vi "ConfigMeasurement.vi"(8 "error in (no error)":errorcluster, 11 "HP3458aDMM in":refnum<class "HP3458aDMM.lvclass">) -> (0 "error out":errorcluster, 3 "HP3458aDMM out":refnum<class "HP3458aDMM.lvclass">)   [LabVIEW 2014, in "SamplerPlugins.lvlib" / "HP3458aDMM.lvclass"]
uses:
  HP3458aDMM.lvclass
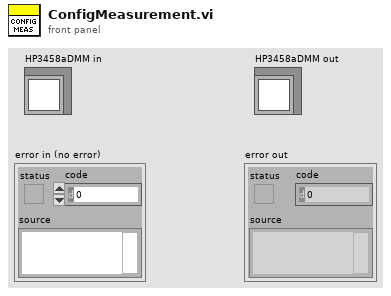
[diagram p1: front panel]
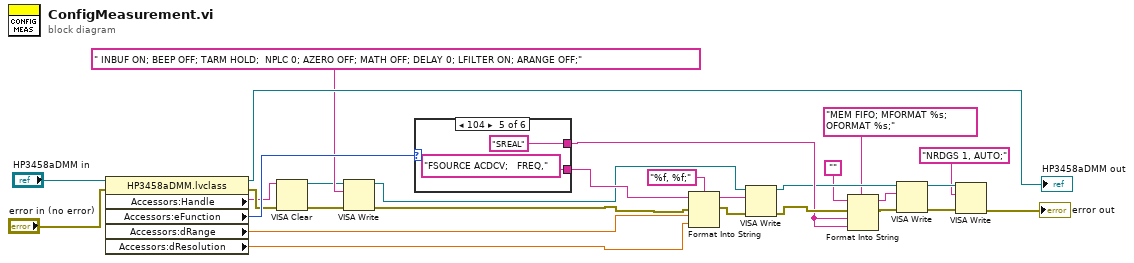
[diagram p0: block diagram]
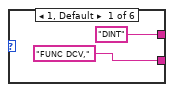
[diagram p2: hidden frame]
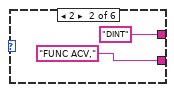
[diagram p3: hidden frame]
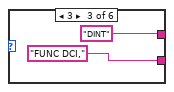
[diagram p4: hidden frame]
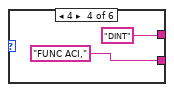
[diagram p5: hidden frame]
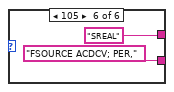
[diagram p6: hidden frame]
diagram:
  n1 = property class="HP3458aDMM.lvclass"(reference="HP3458aDMM in", error in="error in (no error)") -> (reference out=→"HP3458aDMM out":refnum<class "HP3458aDMM.lvclass">, error out=w22:errorcluster, "Accessors:Handle"=w21:string, "Accessors:eFunction"=w23:u16, "Accessors:dRange"=w26:dbl, "Accessors:dResolution"=w25:dbl)
  n2 = VISA Clear(VISA resource name=w21, error in (no error)=w22) -> (VISA resource name out=w12:refnum<visa-resource-name>, error out=w14:errorcluster)
  n3 = VISA Write(VISA resource name=w12, write buffer=" INBUF ON; BEEP OFF; TARM HOLD;  NPLC 0; AZERO OFF; MATH OFF; DELAY 0; LFILTER ON; ARANGE OFF;" ("string"), error in (no error)=w14) -> (VISA resource name out=w11:refnum<visa-resource-name>, error out=w13:errorcluster)  [unwired: 1 out]
  n4 = case shown="104" w23 {
    tunnel: ["FUNC DCV," "FUNC ACV," "FUNC DCI," "FUNC ACI," "FSOURCE ACDCV;   FREQ," "FSOURCE ACDCV; PER,"] -> w16
    tunnel: ["DINT" "DINT" "DINT" "DINT" "SREAL" "SREAL"] -> w8
    frame 1, Default {
    }
    frame 2 {
    }
    frame 3 {
    }
    frame 4 {
    }
    frame 104 {
    }
    frame 105 {
    }
  }
  n5 = Format Into String(format string="%f, %f;", initial string=w16, error in=w13, w26, w25) -> (resulting string=w2:string, error out=w1:errorcluster)
  n6 = VISA Write(VISA resource name=w11, write buffer=w2, error in (no error)=w1) -> (VISA resource name out=w7:refnum<visa-resource-name>, error out=w10:errorcluster)  [unwired: 1 out]
  n7 = Format Into String(format string="MEM FIFO; MFORMAT %s; OFORMAT %s;" ("write buffer"), initial string="", error in=w10, w8, w8) -> (resulting string=w4:string, error out=w9:errorcluster)
  n8 = VISA Write(VISA resource name=w7, write buffer=w4, error in (no error)=w9) -> (VISA resource name out=w20:refnum<visa-resource-name>, error out=w19:errorcluster)  [unwired: 1 out]
  n9 = VISA Write(VISA resource name=w20, write buffer="NRDGS 1, AUTO;", error in (no error)=w19) -> (error out=→"error out":errorcluster)  [unwired: 2 out]
